vi "Utility - Configuration File Generator- Waveform _V1.3.vi"() -> ()   [LabVIEW 2015]
uses:
  <vilib>/LabVIEW Targets/FPGA/cRIO/shared/nicrio_ModuleControls/nicrio_cRIO-9234_DataRatesRing2.ctl
  TDMS Properties.ctl
  <vilib>/LabVIEW Targets/FPGA/cRIO/shared/nicrio_ModuleControls/nicrio_cRIO-9234_ConfigModeRing.ctl
  STA - Waveform V6/Config/Data Rate Conversion.ctl
  Acquisition and Logging Configuration_Waveform - V1.ctl
  <vilib>/Utility/xml.llb/Write to XML File(string).vi
  <vilib>/FTP/NI_FTP.lvlib
panel:
  out "Transmitted to cRIO":bool
  out "unsigned 32bit integer":u32
  out "File Location on host":path
  in  "Data Rate Conversion":T1=[51200.0, 25600.0, 17067.0, 12800.0, 10240.0, 8533.0, 7314.0, 6400.0, 5689.0, 5120.0, 4654.0, 4267.0, 3938.0, 3657.0, 3413.0, 3200.0, 3012.0, 2845.0, 2695.0, 2560.0, 2438.0, 2328.0, 2226.0, 2133.0, 2048.0, 1969.0, 1896.0, 1829.0, 1765.0, 1707.0, 1652.0]
  in  "Repeat Config 1st Raw":bool
  in  "Time Measure (s)":dbl=60.0
  in  "Channel Config":T3(array[cluster])=[{"Channel Name"="mod1/a0\na0\na00\na00", "Sensitivity mV_EU"=1.016, "EU"="ms²", "Input Configuration"=0, "dB Ref EU"=1.0}, {"Channel Name"="mod1/a1", "Sensitivity mV_EU"=1.0, "EU"="V", "Input Configuration"=0, "dB Ref EU"=1.0}, {"Channel Name"="mod1/a2", "Sensitivity mV_EU"=1.0, "EU"="V", "Input Configuration"=0, "dB Ref EU"=1.0}, {"Channel Name"="mod1/a3", "Sensitivity mV_EU"=1.0, "EU"="V", "Input Configuration"=0, "dB Ref EU"=1.0}, {"Channel Name"="mod2/a0", "Sensitivity mV_EU"=1000.0, "EU"="V", "Input Configuration"=0, "dB Ref EU"=1.0}, {"Channel Name"="mod2/a1", "Sensitivity mV_EU"=1000.0, "EU"="V", "Input Configuration"=0, "dB Ref EU"=1.0}, {"Channel Name"="mod2/a2", "Sensitivity mV_EU"=1000.0, "EU"="V", "Input Configuration"=0, "dB Ref EU"=1.0}, {"Channel Name"="mod2/a3", "Sensitivity mV_EU"=1000.0, "EU"="V", "Input Configuration"=0, "dB Ref EU"=1.0}, {"Channel Name"="mod3/a0", "Sensitivity mV_EU"=1000.0, "EU"="V", "Input Configuration"=0, "dB Ref EU"=1.0}, {"Channel Name"="mod3/a1", "Sensitivity mV_EU"=1000.0, "EU"="V", "Input Configuration"=0, "dB Ref EU"=1.0}, {"Channel Name"="mod3/a2", "Sensitivity mV_EU"=1000.0, "EU"="V", "Input Configuration"=0, "dB Ref EU"=1.0}, {"Channel Name"="mod3/a3", "Sensitivity mV_EU"=1000.0, "EU"="V", "Input Configuration"=0, "dB Ref EU"=1.0}, {"Channel Name"="mod4/a0", "Sensitivity mV_EU"=1000.0, "EU"="V", "Input Configuration"=0, "dB Ref EU"=1.0}, {"Channel Name"="mod4/a1", "Sensitivity mV_EU"=1000.0, "EU"="V", "Input Configuration"=0, "dB Ref EU"=1.0}, {"Channel Name"="mod4/a2", "Sensitivity mV_EU"=1000.0, "EU"="V", "Input Configuration"=0, "dB Ref EU"=1.0}, {"Channel Name"="mod4/a3", "Sensitivity mV_EU"=1000.0, "EU"="V", "Input Configuration"=0, "dB Ref EU"=1.0}] caption="Channel Name      Sensitivity [mV/EU]              EU                           dB Ref [EU]                Input Typ" {"Input Configuration" items=["AC Coupled", "DC Coupled", "IEPE AC Coupled"]}
  in  "TDMS Properties":T4[](array[typedef])=[{"Name"="Enterprise", "Value"="[CompanyName]"}, {"Name"="Author", "Value"="[DeveloperName]"}, {"Name"="Operator", "Value"="[OperatorName]"}, {"Name"="TestSystem", "Value"="[SystemName]"}, {"Name"="Site", "Value"="[Location]"}, {"Name"="Line", "Value"="[Line]"}, {"Name"="Machine", "Value"="[MachineName]"}, {"Name"="Description", "Value"="[Description]"}]
  in  "Trigger - Time (Minute)":i32=30
  in  "Trigger - Channel":i32
  in  "Trigger - RMS Value":dbl=1.8
  in  "Number of Channels":i32=16
  in  "Data File Name":string="cRIO_Data"
  in  "Samples per Read":i32=12800
  in  "Data Rate":T5=1 items=["51.200 kS/s (NI 9234)"=1, "25.600 kS/s (NI 9234)"=2, "17.067 kS/s (NI 9234)"=3, "12.800 kS/s (NI 9234)"=4, "10.240 kS/s (NI 9234)"=5, "8.533 kS/s (NI 9234)"=6, "7.314 kS/s (NI 9234)"=7, "6.400 kS/s (NI 9234)"=8, "5.689 kS/s (NI 9234)"=9, "5.120 kS/s (NI 9234)"=10, "4.654 kS/s (NI 9234)"=11, "4.267 kS/s (NI 9234)"=12, "3.938 kS/s (NI 9234)"=13, "3.657 kS/s (NI 9234)"=14, "3.413 kS/s (NI 9234)"=15, "3.200 kS/s (NI 9234)"=16, "3.012 kS/s (NI 9234)"=17, "2.845 kS/s (NI 9234)"=18, "2.695 kS/s (NI 9234)"=19, "2.560 kS/s (NI 9234)"=20, "2.438 kS/s (NI 9234)"=21, "2.328 kS/s (NI 9234)"=22, "2.226 kS/s (NI 9234)"=23, "2.133 kS/s (NI 9234)"=24, "2.048 kS/s (NI 9234)"=25, "1.969 kS/s (NI 9234)"=26, "1.896 kS/s (NI 9234)"=27, "1.829 kS/s (NI 9234)"=28, "1.765 kS/s (NI 9234)"=29, "1.707 kS/s (NI 9234)"=30, "1.652 kS/s (NI 9234)"=31]
  # "Instructions: Populate the controls below with desired values, then run the VI to generate a 'Config.xml' file in the root folder of your project.  \n\nNote:  Once you have generated the Config.xml file, you will need to copy it to the root folder of your RT Target."
  # "Channels"
  # "Acquisition"
  # "Logging"
  # "Trigger"
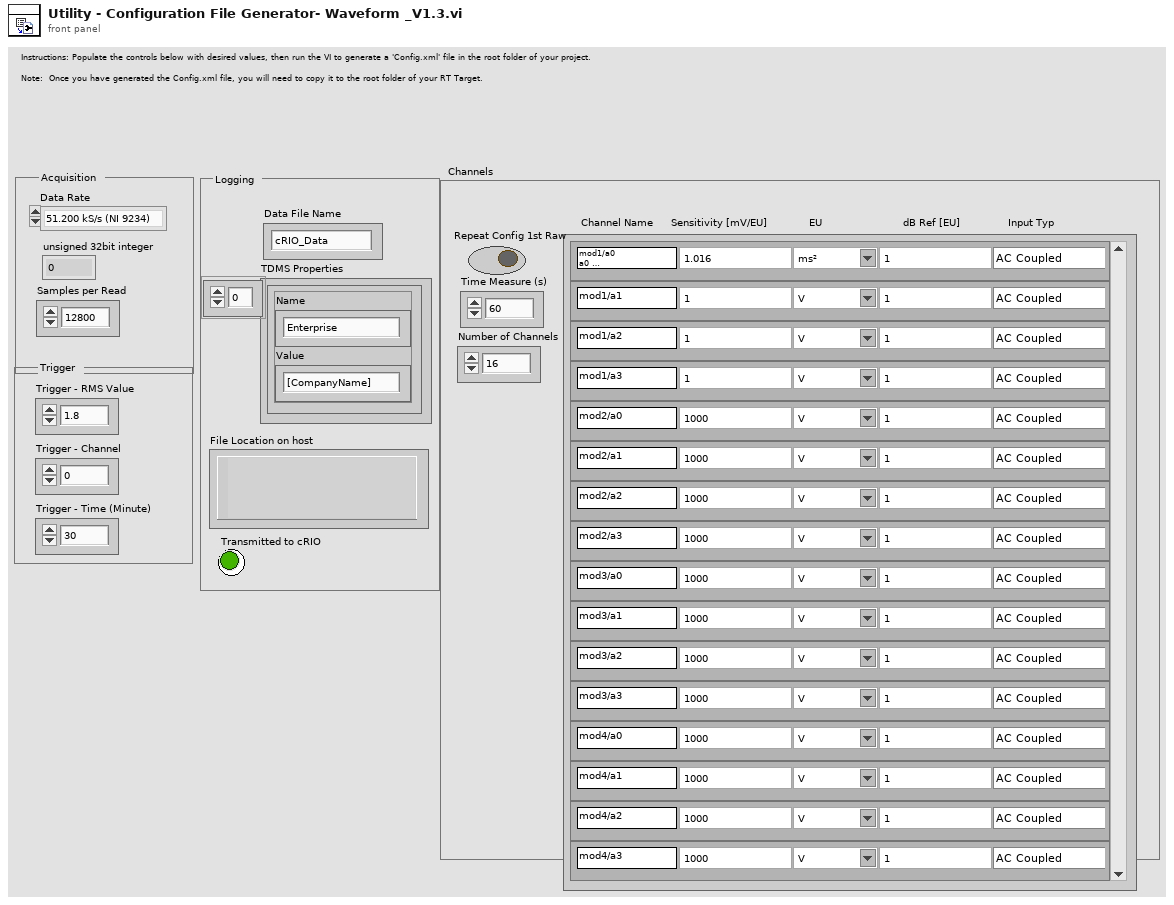
[diagram p1: front panel]
types:
  T1 = typedef "Data Rate Conversion.ctl" = dbl[]
  T2 = typedef "nicrio_cRIO-9234_ConfigModeRing.ctl" = u8
  T3 = cluster{"Channel Name":string, "Sensitivity mV_EU":dbl, "EU":string, "Input Configuration":T2, "dB Ref EU":dbl}[]
  T4 = typedef "TDMS Properties.ctl" = cluster{"Name":string, "Value":string}
  T5 = typedef "nicrio_cRIO-9234_DataRatesRing2.ctl" = u8
  T6 = typedef "Acquisition and Logging Configuration_Waveform - V1.ctl" = cluster{"Samples per Read":i32, "Number of Reads to Save":i32, "Data File Name":string, "TDMS Properties":T4[], "Number of Channels":i32, "Trigger - RMS Value":dbl, "Trigger - Channel":i32, "Trigger - Time (Minute)":i32, "Channel Config":cluster{"Channel Name":string, "Sensitivity mV_EU":dbl, "EU":string, "Input Configuration":T2, "dB Ref EU":dbl}[], "data rate (S/s)":u32, "Time Measure":dbl}
  T7 = cluster{"Channel Name":string, "Sensitivity mV_EU":dbl, "EU":string, "Input Configuration":T2, "dB Ref EU":dbl}
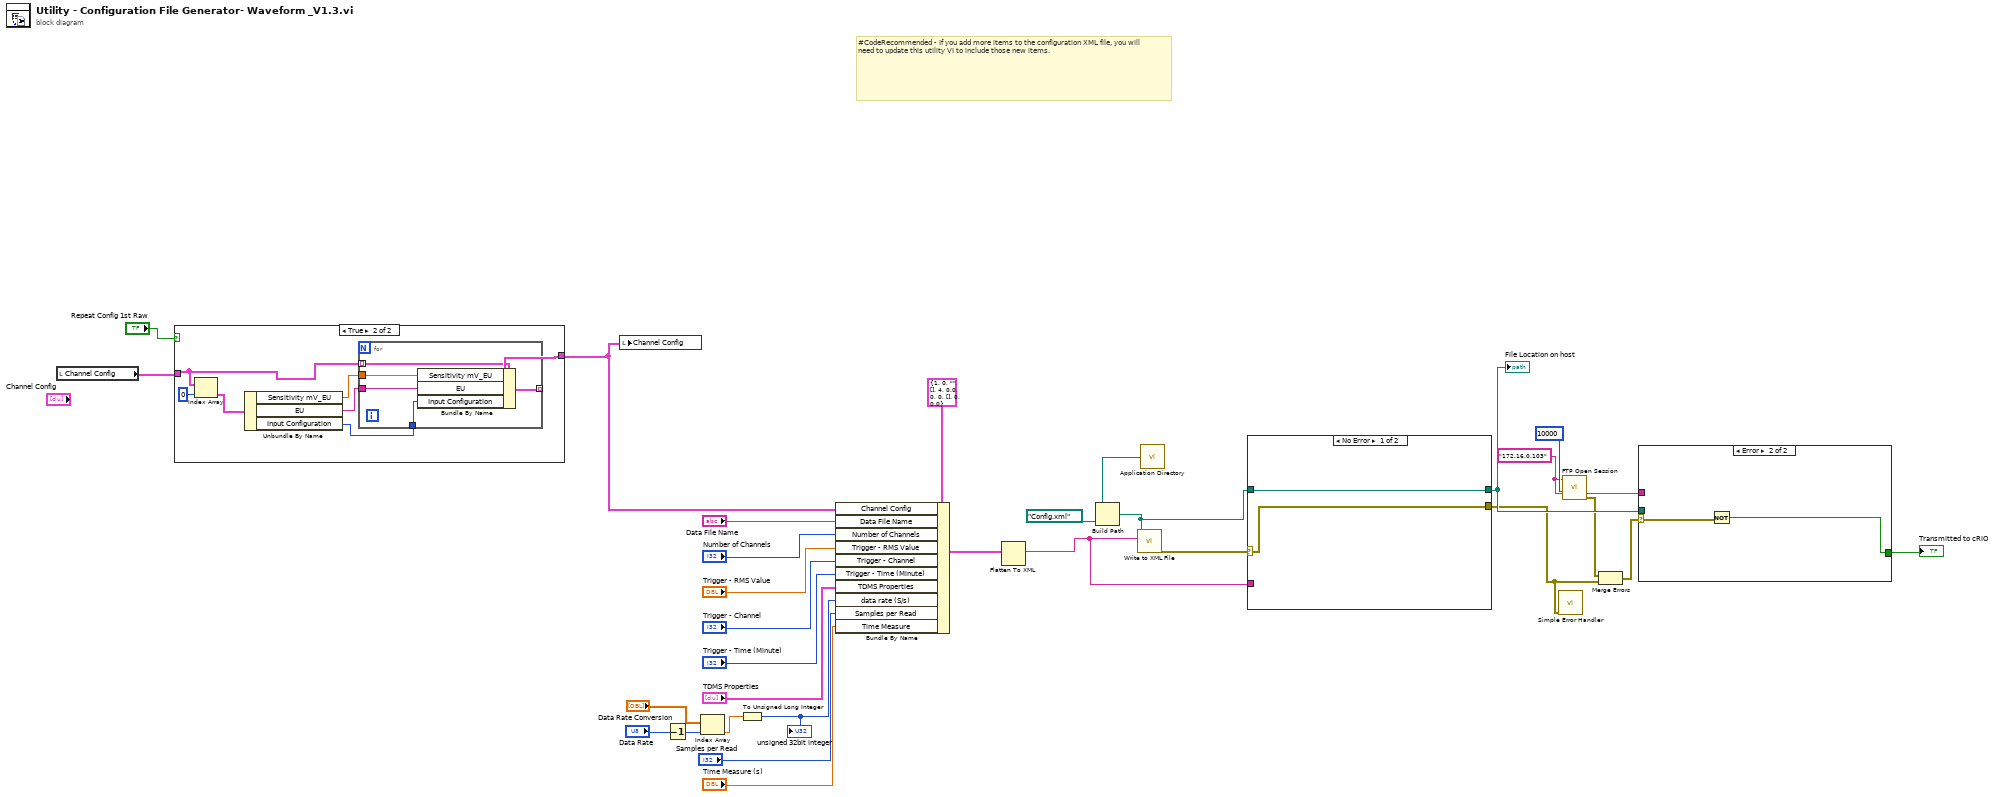
[diagram p0: block diagram]
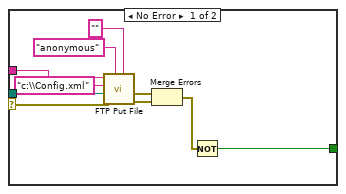
[diagram p2: hidden frame]
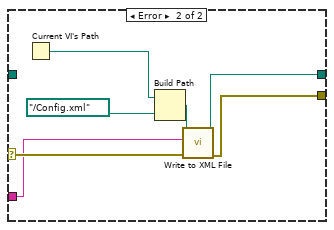
[diagram p3: hidden frame]
diagram:
  w7 = "172.16.0.103" ("address")
  # "#CodeRecommended - If you add more items to the configuration XML file, you will need to update this utility VI to include those new items."
  n1 = local read "Channel Config"() -> (w20:T3)
  n2 = case shown="True" "Repeat Config 1st Raw" {
    tunnel: w20 -> [w31 w32]
    tunnel: [w31 w33] -> w19
    frame False {
    }
    frame True {
      n3 = Index Array(array=w32, index=0) -> (element=w37:T7)
      n4 = Unbundle By Name(w37) -> ("Sensitivity mV_EU"=w36:dbl, "EU"=w35:string, "Input Configuration"=w34:T2)
      n5 = for {
        tunnel: w32 -> [w39] mode=indexing
        tunnel: w36 -> [w43]
        tunnel: w35 -> [w42]
        tunnel: w34 -> [w41]
        tunnel: [w40] -> w33 mode=indexing
        n6 = Bundle By Name(cluster=w39, "Sensitivity mV_EU"=w43, "EU"=w42, "Input Configuration"=w41) -> (w40:T7)
      }
    }
  }
  n7 = local write "Channel Config"(w19) -> ()
  n8 = Decrement(x="Data Rate") -> (x-1=w17:T5)
  n9 = Index Array(array="Data Rate Conversion", index=w17) -> (element=w16:dbl)
  n10 = To Unsigned Long Integer(number=w16) -> (unsigned 32bit integer=w15:u32)
  "unsigned 32bit integer" <- w15
  n11 = Bundle By Name(cluster=T6 {"Samples per Read"=1, "Number of Reads to Save"=0, "Data File Name"="", "TDMS Properties"=[], "Number of Channels"=4, "Trigger - RMS Value"=0.0, "Trigger - Channel"=0, "Trigger - Time (Minute)"=0, "Channel Config"=[], "data rate (S/s)"=0, "Time Measure"=0.0} ("Acquisition and Logging Configuration"), "Channel Config"=w19, "Data File Name"="Data File Name", "Number of Channels"="Number of Channels", "Trigger - RMS Value"="Trigger - RMS Value", "Trigger - Channel"="Trigger - Channel", "Trigger - Time (Minute)"="Trigger - Time (Minute)", "TDMS Properties"="TDMS Properties", "data rate (S/s)"=w15, "Samples per Read"="Samples per Read", "Time Measure"="Time Measure (s)") -> (w23:T6)
  n12 = Flatten To XML(anything=w23) -> (xml string=w10:string)
  n13 = call <vilib>:"Application Directory.vi"() -> ("Application Directory"=w4:path)
  n14 = Build Path(base path=w4, name or relative path=path "Config.xml") -> (appended path=w3:path)
  n15 = call-poly <vilib>:"Write to XML File.vi"("XML Input"=w10, "XML File Path"=w3) -> ("error out"=w11:errorcluster)  [unwired: 7 in, 2 out]
  n16 = case shown="No Error" w11 {
    selector: w11 -> [w45 w51]
    tunnel: w10 -> [_ w50]
    tunnel: [w45 w49] -> w2
    tunnel: [w44 w46] -> w8
    tunnel: w3 -> [w44 _]
    frame No Error {
    }
    frame Error {
      n17 = Current VI's Path() -> (path=w47:path)
      n18 = Build Path(base path=w47, name or relative path=path "../Config.xml") -> (appended path=w48:path)
      n19 = call-poly <vilib>:"Write to XML File.vi"("error in (no error)"=w51, "XML Input"=w50, "XML File Path"=w48) -> ("error out"=w49:errorcluster, "XML File Path(duplicate)"=w46:path)  [unwired: 6 in, 1 out]
    }
  }
  "File Location on host" <- w8
  n20 = call <vilib>:"Simple Error Handler.vi"("error in (no error)"=w2) -> ()  [unwired: 4 in, 5 out]
  n21 = call <vilib>:"FTP Open Session.vi"("timeout ms (60000)"=10000, "address"=w7) -> ("error out"=w6:errorcluster)  [unwired: 6 in, 3 out]
  n22 = Merge Errors(w6, w2) -> (w5:errorcluster)
  n23 = case shown="Error" w5 {
    selector: w5 -> [w55 w64]
    tunnel: w8 -> [w62 _]
    tunnel: w7 -> [w61 _]
    tunnel: [w53 w63] -> w1
    frame No Error {
      n24 = call <vilib>:"FTP Put File.vi"("password"="", "user"="anonymous", "error in (no error)"=w55, "local path"=w62, "remote path"="c:\\Config.xml", "host"=w61) -> ("error out"=w56:errorcluster, "file error"=w57:errorcluster)  [unwired: 4 in]
      n25 = Merge Errors(w57, w56) -> (w54:errorcluster)
      n26 = Not(x=w54) -> (.not. x?=w53:bool)
    }
    frame Error {
      n27 = Not(x=w64) -> (.not. x?=w63:bool)
    }
  }
  "Transmitted to cRIO" <- w1
